vi "Config to JSON.vi"(8 "error in (no error)":errorcluster, 11 "Auto Vision Config":T1={"RIO Device"="PXI1Slot4", "Serial Channel"="SI0", "SERDES Script"="C:\\dev\\ttashjia\\GSE\\GSE_1486_4in4out\\Host\\Scripts\\DS90UB954\\Acq\\Loopback.py", "POC Source"=0, "CSI-2 Data Source"=1, "Lane Count"=4, "Reference Clock"=25000000.0, "Image Data Type"=44, "Interpretation"=1, "Pattern"=0, "Algorithm"=0, "Virtual Channel"=0, "Embedded Data"={"Pre-embedded Lines"=4.0, "Pre-embedded Line Length"=1920.0, "Post-embedded Lines"=2.0, "Post-embedded Line Length"=1920.0, "Frame Count"={"Line"=0.0, "Offset"=2.0, "Byte Count"=4.0}}, "Registers"=[{"Name"="Temp0", "Device"=97, "Address"=27, "Min"=0, "Max"=16}, {"Name"="Temp1", "Device"=97, "Address"=90, "Min"=0, "Max"=16}], "Log Path"="C:\\data"}) -> (0 "error out":errorcluster, 3 "JSON string":string="{\n  \"RIO Device\":\"PXI1Slot4\",\n  \"Serial Channel\":\"SI0\",\n  \"SERDES Script\":\"C:\\\\dev\\\\ttashjia\\\\GSE\\\\GSE_1486_4in4out\\\\Host\\\\Scripts\\\\DS90UB954\\\\Acq\\\\Loopback.py\",\n  \"POC Source\":0,\n  \"CSI-2 Data Source\":1,\n  \"Lane Count\":4,\n  \"Reference Clock\":25000000,\n  \"Image Data Type\":44,\n  \"Interpretation\":1,\n  \"Pattern\":0,\n  \"Algorithm\":0,\n  \"Virtual Channel\":0,\n  \"Embedded Data\":{\n    \"Pre-embedded Lines\":4,\n    \"Pre-embedded Line Length\":1920,\n    \"Post-embedded Lines\":2,\n    \"Post-embedded Line Length\":1920,\n    \"Frame Count\":{\"Line\":0,\"Offset\":2,\"Byte Count\":4}\n  },\n  \"Registers\":[\n    {\n      \"Name\":\"Temp0\",\n      \"Device\":97,\n      \"Address\":27,\n      \"Min\":0,\n      \"Max\":16\n    },\n    {\n      \"Name\":\"Temp1\",\n      \"Device\":97,\n      \"Address\":90,\n      \"Min\":0,\n      \"Max\":16\n    }\n  ],\n  \"Log Path\":\"C:\\\\data\"\n}")   [LabVIEW 2025, in "Automotive Vision UI.lvlib"]
uses:
  Automotive Vision UI.lvlib
  auto vision config.ctl
  register.ctl
  <vilib>/JDP Science/JSONtext/JSONtext.lvlib
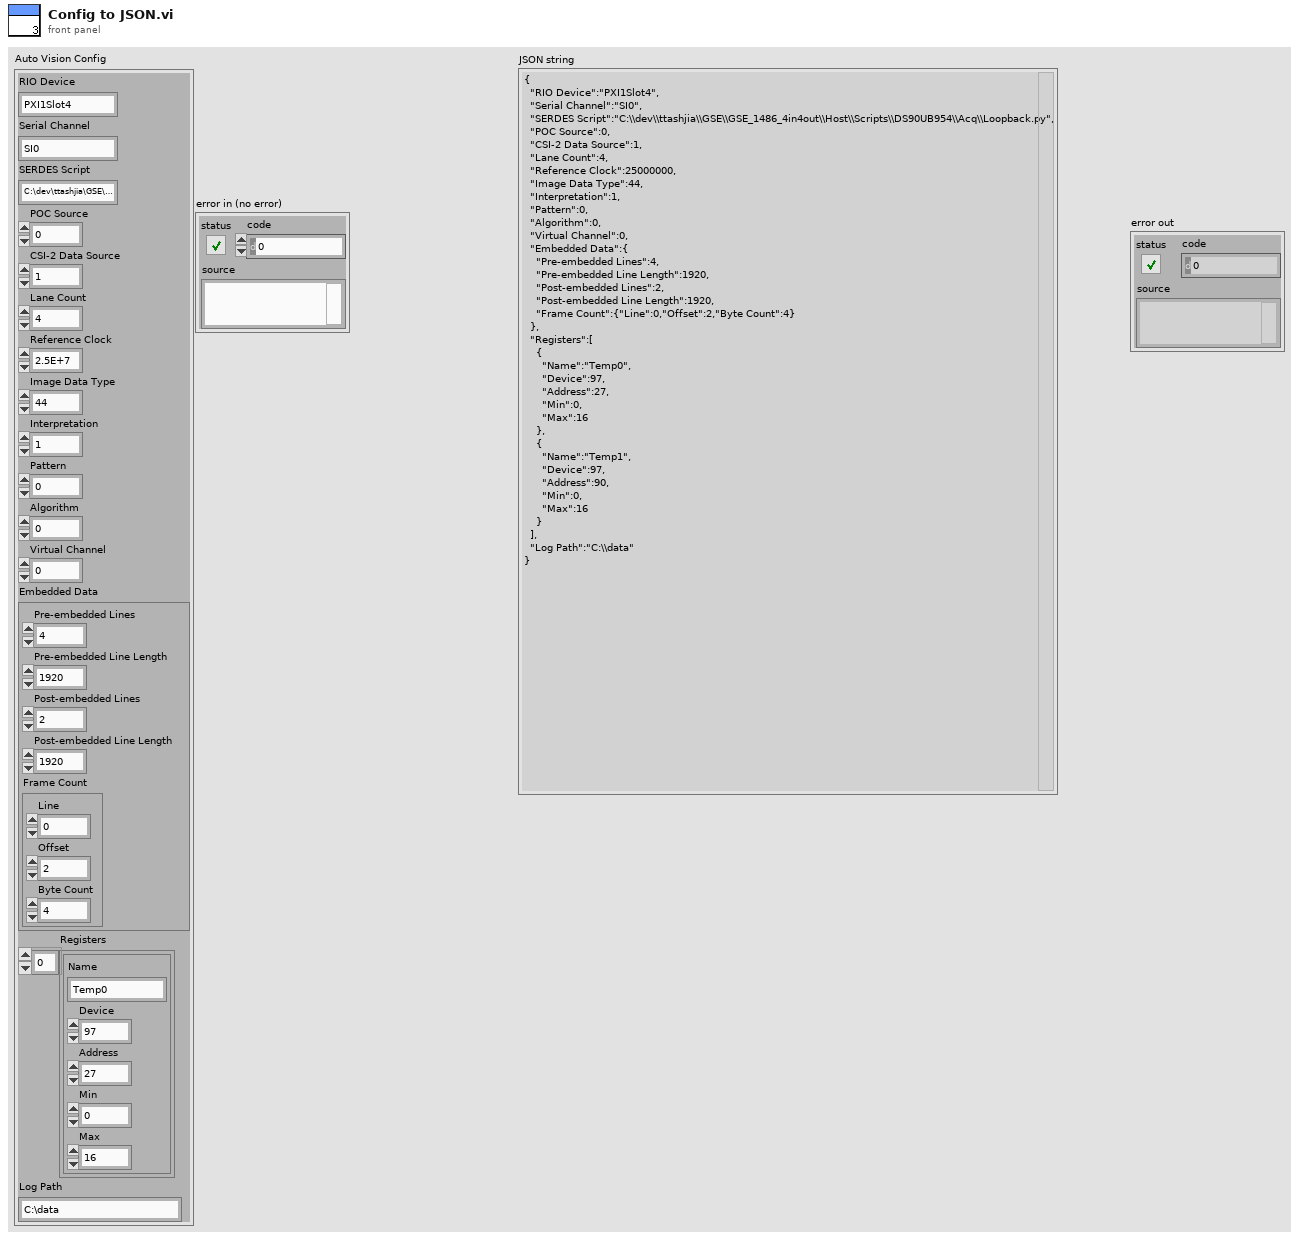
[diagram p1: front panel]
types:
  T1 = typedef "Automotive Vision UI.lvlib/auto vision config.ctl" = cluster{"RIO Device":string, "Serial Channel":string, "SERDES Script":string, "POC Source":u32, "CSI-2 Data Source":u32, "Lane Count":u32, "Reference Clock":dbl, "Image Data Type":u32, "Interpretation":u32, "Pattern":u32, "Algorithm":u32, "Virtual Channel":u32, "Embedded Data":cluster{"Pre-embedded Lines":dbl, "Pre-embedded Line Length":dbl, "Post-embedded Lines":dbl, "Post-embedded Line Length":dbl, "Frame Count":cluster{"Line":dbl, "Offset":dbl, "Byte Count":dbl}}, "Registers":T2[], "Log Path":string}
  T2 = typedef "Automotive Vision UI.lvlib/register.ctl" = cluster{"Name":string, "Device":u8, "Address":u16, "Min":u16, "Max":u16}
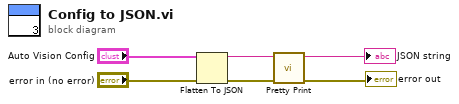
[diagram p0: block diagram]
diagram:
  n1 = Flatten To JSON(anything="Auto Vision Config", error in (no error)="error in (no error)") -> (JSON string=w3:string, 11:w4:errorcluster)  [unwired: 1 in]
  n2 = call <vilib>:"Pretty Print.vi"("error in (no error)"=w4, "JSON"=w3) -> ("error out"=→"error out":errorcluster, "<JSON>"=→"JSON string":string)  [unwired: 7 in, 1 out]
